vi "Update from Module Class.vi"(8 "error in":errorcluster, 9 "module in":refnum<class "Module.lvclass">, 10 "slot ref in":T1=18446744073709551615 format="%.0x", 11 "SD Module in":refnum<class "SD Module.lvclass">) -> (0 "error out":errorcluster, 1 "module out":refnum<class "Module.lvclass">, 2 "slot ref out":T1=18446744073709551615 format="%.0x", 3 "SD Module out":refnum<class "SD Module.lvclass">)   [LabVIEW 2017, in "Modules.lvlib" / "SD Module.lvclass"]
uses:
  SD Module.lvclass
  niveristand-scan-engine-ethercat-custom-device/Custom Device Source/Scripting/Modules/Module/Module.lvclass
  <vilib>/NI Veristand/Custom Device API/Custom Device Item Ref.ctl
  niveristand-scan-engine-ethercat-custom-device/Custom Device Source/Scripting/Modules/Mode Classes/Mode/Mode.lvclass
  RSI Module/RSI Module.lvclass
  <vilib>/NI Veristand/Custom Device API/Custom Device API.lvlib
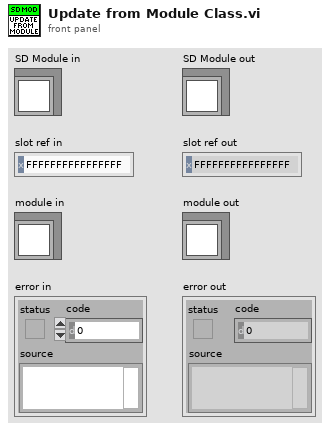
[diagram p1: front panel]
types:
  T1 = typedef "Custom Device API.lvlib/Custom Device Item Ref.ctl" = u64
  T2 = cluster{"PWM Channels":cluster{"PWM frequency":u32}[]}
  T3 = cluster{"Drive From Slot":u32, "CDO Channels":cluster{"Counter driven enabled":bool}[]}
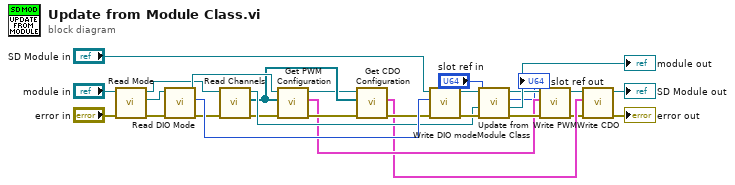
[diagram p0: block diagram]
diagram:
  n1 = call-dynamic "Read Mode.vi"("error in"="error in", "module in"="module in") -> ("error out"=w24:errorcluster, "mode"=w25:refnum<class "Mode.lvclass">, "module out"=w17:refnum<class "Module.lvclass">)  [unwired: 7 in]
  n2 = call-dynamic "Read DIO Mode.vi"("error in"=w24, "mode in"=w25) -> ("error out"=w18:errorcluster, "DIO mode"=w23:u32, "mode out"=w19:refnum<class "Mode.lvclass">)  [unwired: 7 in]
  n3 = call-dynamic "Read Channels.vi"("error in"=w18, "module in"=w17) -> ("error out"=w15:errorcluster, "channels"=w13:refnum<class "Channel.lvclass">[], "module out"=w16:refnum<class "Module.lvclass">)  [unwired: 7 in]
  n4 = call-dynamic "Get PWM Configuration.vi"("error in"=w15, "channels"=w13, "mode in"=w19) -> ("error out"=w14:errorcluster, "PWM"=w8:T2, "mode out"=w12:refnum<class "Mode.lvclass">)  [unwired: 6 in]
  n5 = call-dynamic "Get CDO Configuration.vi"("error in"=w14, "channels"=w13, "mode in"=w12) -> ("error out"=w11:errorcluster, "CDO"=w6:T3)  [unwired: 6 in, 1 out]
  n6 = call-dynamic "Write DIO mode.vi"("error in (no error)"=w11, "DIO mode"=w23, "SD Module in"="SD Module in") -> ("error out"=w21:errorcluster, "SD Module out"=w20:refnum<class "SD Module.lvclass">)  [unwired: 7 in]
  n7 = call-parent "Update from Module Class.vi"("error in"=w21, "module in"=w16, "slot ref in"="slot ref in", "RSI Module in"=w20) -> ("error out"=w10:errorcluster, "module out"=→"module out":refnum<class "Module.lvclass">, "slot ref out"=→"slot ref out":T1, "RSI Module out"=w9:refnum<class "SD Module.lvclass">)  [unwired: 4 in]
  n8 = call-dynamic "Write PWM.vi"("error in (no error)"=w10, "PWM"=w8, "SD Module in"=w9) -> ("error out"=w5:errorcluster, "SD Module out"=w7:refnum<class "SD Module.lvclass">)  [unwired: 7 in]
  n9 = call-dynamic "Write CDO.vi"("error in (no error)"=w5, "CDO"=w6, "SD Module in"=w7) -> ("error out"=→"error out":errorcluster, "SD Module out"=→"SD Module out":refnum<class "SD Module.lvclass">)  [unwired: 7 in]
